vi "Launch Actor.vi"(8 "error in (no error)":errorcluster, 10 "Show Front Panel? (F)":bool, 11 "Actor Interface in":refnum<data-value>) -> (0 "error out":errorcluster, 1 "Actor Already Launched":bool, 3 "Actor Interface out":refnum<data-value>)   [LabVIEW 2018, in "Actor.lvlib" / "Actor-Interface.lvclass"]
uses:
  Actor-Interface.lvclass
  Actor-Interface.lvclass/Actor-Interface.ctl
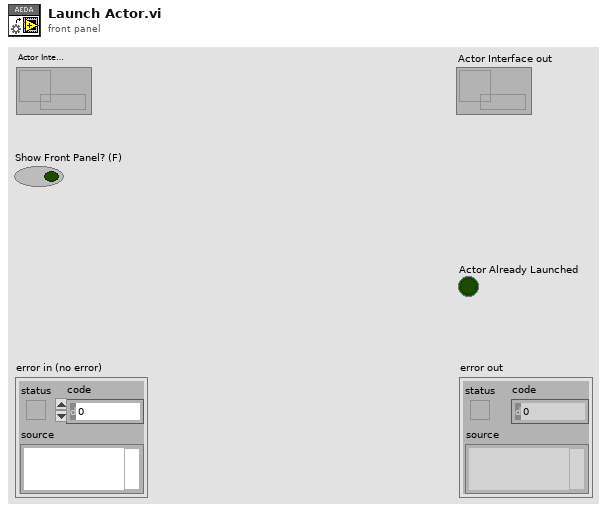
[diagram p1: front panel]
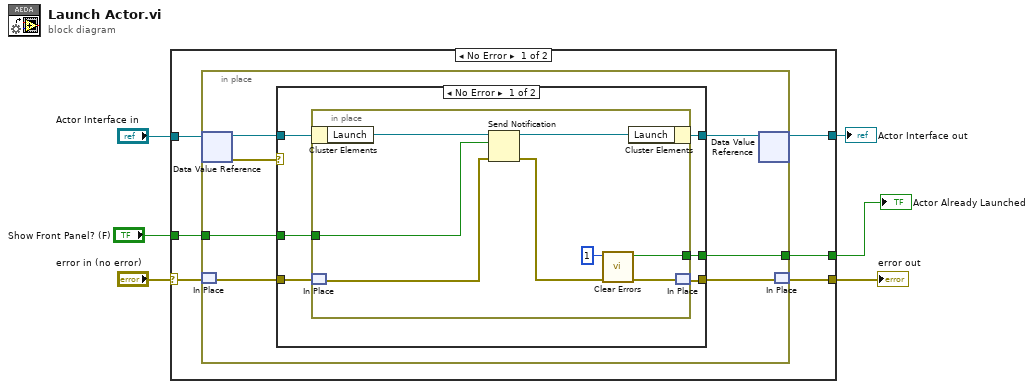
[diagram p0: block diagram]
diagram:
  n1 = case shown="No Error" "error in (no error)" {
    selector: "error in (no error)" -> [w11 w37]
    tunnel: [w10 w37] -> w5
    tunnel: [w9 w36] -> w1
    tunnel: "Actor Interface in" -> [w12 w36]
    tunnel: [w8 _] -> w3
    tunnel: "Show Front Panel? (F)" -> [w7 _]
    frame No Error {
      n2 = in-place {
        in-place-border: [w14] -> w8
        in-place-border: w7 -> [w13]
        n3 = in-place-dvr #1(w12) -> (w18:refnum<class "Actor-Interface.lvclass">, w19:errorcluster)
        n4 = in-place-match #2(w11) -> (w16:errorcluster)
        n5 = case shown="No Error" w19 {
          selector: w19 -> [_ w35]
          tunnel: w18 -> [w25 w34]
          tunnel: [w22 w34] -> w17
          tunnel: w16 -> [w24 _]
          tunnel: [w23 w35] -> w15
          tunnel: [w21 _] -> w14
          tunnel: w13 -> [w20 _]
          frame No Error {
            n6 = in-place {
              in-place-border: [w27] -> w21
              in-place-border: w20 -> [w26]
              n7 = in-place-cluster #3(w25) -> ("Launch"=w33:refnum<notifier>)
              n8 = in-place-match #4(w24) -> (w32:errorcluster)
              n9 = Send Notification(notification=w26, notifier=w33, error in (no error)=w32) -> (notifier out=w31:refnum<notifier>, error out=w30:errorcluster)
              n10 = call <vilib>:"Clear Errors.vi"("error in (no error)"=w30, "specific error code to clear (0: all)"=1) -> ("error out"=w29:errorcluster, "specific error cleared?"=w27:bool)  [unwired: 4 in]
              n11 = in-place-cluster #3("Launch"=w31) -> (w22:refnum<class "Actor-Interface.lvclass">)
              n12 = in-place-match #4(w29) -> (w23:errorcluster)
            }
          }
          frame Error {
          }
        }
        n13 = in-place-dvr #1(w17) -> (w9:refnum<data-value>)  [unwired: 1 out]
        n14 = in-place-match #2(w15) -> (w10:errorcluster)
      }
    }
    frame Error {
    }
  }
  "error out" <- w5
  "Actor Already Launched" <- w3
  "Actor Interface out" <- w1
